vi "calcualte_scens.vi"(3 "Sort Scen":bool=TRUE, 5 "vy_in":T2(array[cluster])) -> (0 "boundaries":T1(array[cluster]), 2 "Scen out":T3(array[cluster]) {"xy_k_value" format="%#_3f"; "polygon" format="%#_3f"})   [LabVIEW 2011]
panel:
  out "scen_out":picture
  out "vy_in":picture
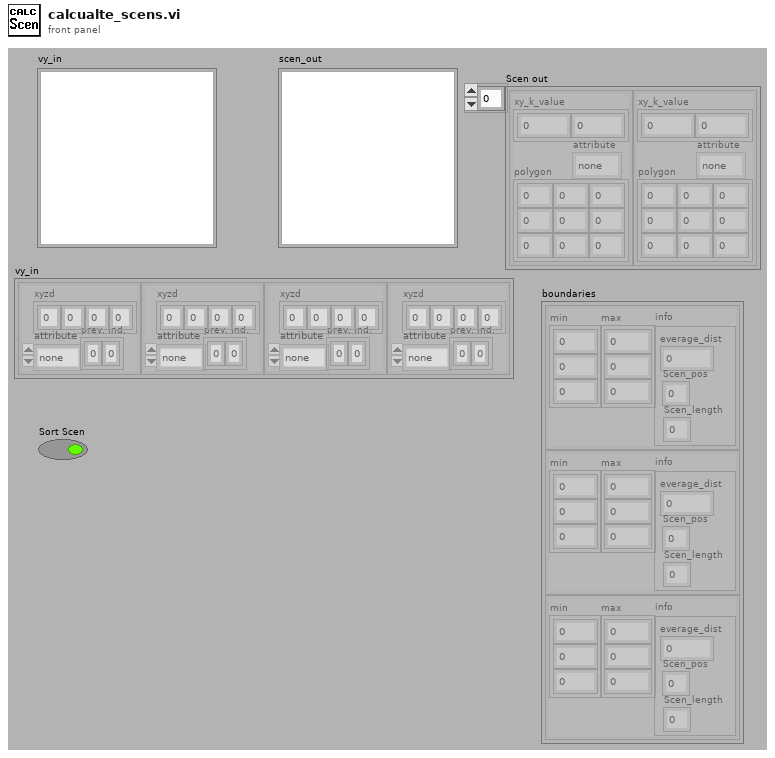
[diagram p1: front panel]
types:
  T1 = cluster{"min":dbl[], "max":dbl[], "info":cluster{"everage_dist":dbl, "Scen_pos":u16, "Scen_length":u16}}[]
  T2 = cluster{"xyzd":dbl[], "attribute":enum16{"none", "transparent", "reflective", "white", "black", "grey", "red", "yellow", "green", "blue", "pink"}, "prev. Ind.":i16[]}[]
  T3 = cluster{"xy_k_value":dbl[], "polygon":dbl[][], "attribute":enum16{"none", "transparent", "reflective", "white", "black", "grey", "red", "yellow", "green", "blue", "pink"}}[]
  T4 = cluster{"min":dbl[], "max":dbl[], "info":cluster{"everage_dist":dbl, "scen_pos":u16, "scen_length":u16}}
  T5 = cluster{"xy_k_value":dbl[], "polygon":dbl[][], "attribute":enum16{"none", "transparent", "reflective", "white", "black", "grey", "red", "yellow", "green", "blue", "pink"}}
  T6 = cluster{"min":dbl[], "max":dbl[], "info":cluster{"everage_dist":dbl, "scen_pos":u16, "scen_length":u16}}[]
  T7 = enum16{"none", "transparent", "reflective", "white", "black", "red", "yellow", "green", "blue", "pink"}
  T8 = enum16{"none", "transparent", "reflective", "white", "black", "grey", "red", "yellow", "green", "blue", "pink"}
  T9 = cluster{"xyzd":dbl[], "attribute":enum16{"none", "transparent", "reflective", "white", "black", "grey", "red", "yellow", "green", "blue", "pink"}, "prev. Ind.":i16[]}
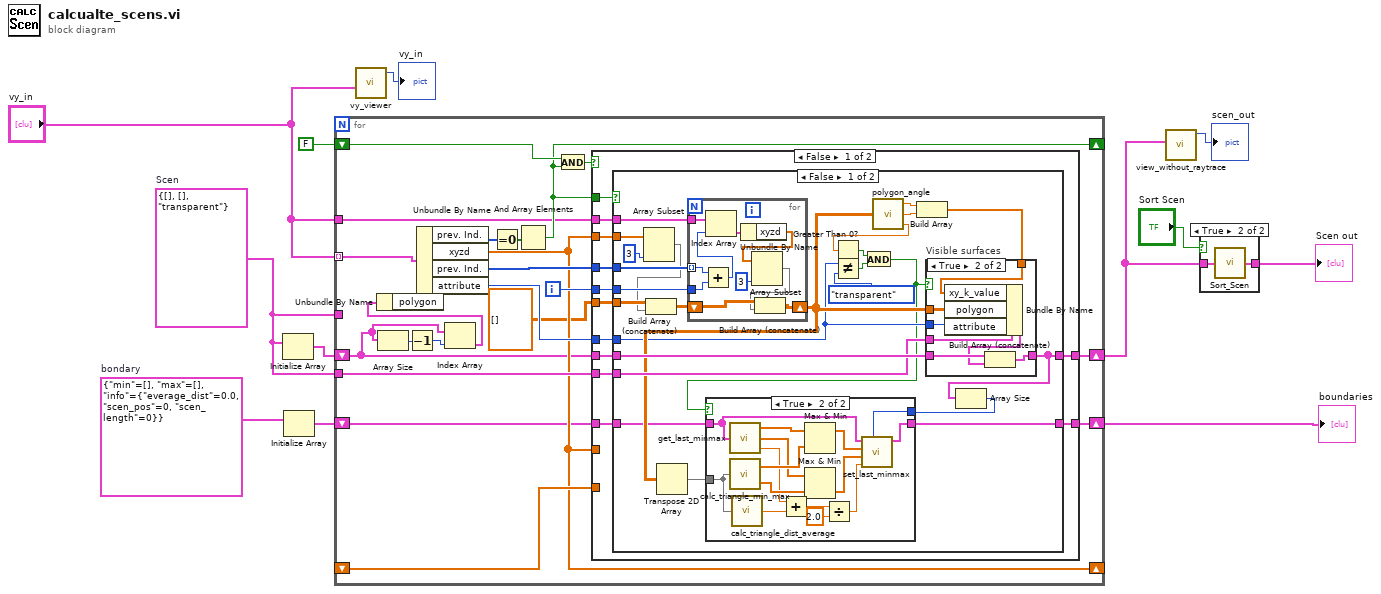
[diagram p0: block diagram]
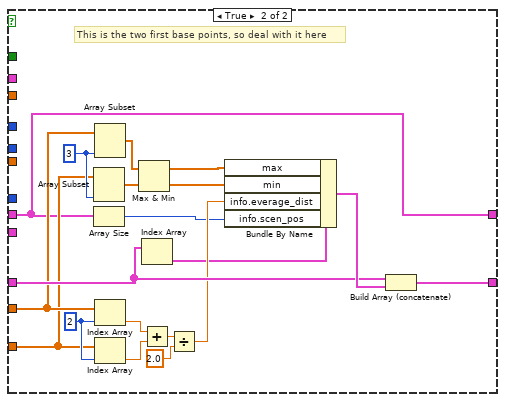
[diagram p6: hidden frame]
diagram:
  w6 = T4 {"min"=[], "max"=[], "info"={"everage_dist"=0.0, "scen_pos"=0, "scen_length"=0}}  # bondary
  w10 = T5 {"xy_k_value"=[], "polygon"=[], "attribute"=enum."transparent"}  # Scen
  n1 = Initialize Array(w10) -> (w9:T3)  [unwired: 1 in]
  n2 = Initialize Array(w6) -> (w7:T6)  [unwired: 1 in]
  n3 = for {
    tunnel: "vy_in" -> [w33] mode=indexing
    shift-right: [w13] -> w5
    shift-left: w7 -> [w14]
    shift-right: [w27] -> _
    shift-left: FALSE -> [w28]
    shift-right: [w18] -> _
    shift-left: _ -> [w29]
    shift-right: [w22] -> w2
    shift-left: w9 -> [w17]
    tunnel: "vy_in" -> [w24]
    tunnel: w10 -> [_]
    tunnel: w10 -> [w23]
    i -> [w25]
    n4 = Array Size(array=w17) -> (size(s)=w20:i32)
    n5 = Decrement(x=w20) -> (x-1=w19:i32)
    n6 = Unbundle By Name(w33) -> ("prev. Ind."=w32:i16[], "xyzd"=w18:dbl[], "prev. Ind."=w26:i16[], "attribute"=w21:T8)
    n7 = Index Array(array=w17, index=w19) -> (element=w16:T5)
    n8 = Unbundle By Name(w16) -> ()  [unwired: 1 out]
    n9 = Equal To 0?(x=w32) -> (x = 0?=w31:bool[])
    n10 = And Array Elements(Boolean array=w31) -> (logical AND=w27:bool)
    n11 = And(x=w28, y=w27) -> (x .and. y?=w30:bool)
    n12 = case shown="False" w30 {
      tunnel: w14 -> [w36 w114]
      tunnel: [w34 w109] -> w13
      tunnel: w18 -> [_ w113]
      tunnel: w29 -> [_ w111]
      tunnel: w27 -> [w45 _]
      tunnel: dbl[][] [] ("polygon") -> [w44 _]
      tunnel: w26 -> [w43 _]
      tunnel: w25 -> [w42 _]
      tunnel: w24 -> [w41 _]
      tunnel: w18 -> [w40 _]
      tunnel: w17 -> [w39 w108]
      tunnel: w23 -> [w38 _]
      tunnel: [w37 w108] -> w22
      tunnel: w21 -> [w35 _]
      frame False {
        n13 = case shown="False" w45 {
          tunnel: w44 -> [w60 _]
          tunnel: w43 -> [w70 _]
          tunnel: w42 -> [w69 _]
          tunnel: w41 -> [w68 _]
          tunnel: w40 -> [w61 _]
          tunnel: w39 -> [w66 w106]
          tunnel: w38 -> [w65 _]
          tunnel: [w55 w106] -> w37
          tunnel: w36 -> [w49 w105]
          tunnel: [w48 w105] -> w34
          tunnel: w35 -> [w51 _]
          frame False {
            n14 = Array Subset(array=w61, length=3) -> (w59:dbl[])  [unwired: 1 in]
            n15 = Build Array (concatenate)(w60, w59) -> (w58:dbl[][])
            n16 = for {
              tunnel: w70 -> [w104] mode=indexing
              tunnel: w69 -> [w103]
              tunnel: w68 -> [w102]
              shift-right: [w95] -> w57
              shift-left: w58 -> [w97]
              n17 = Add(x=w104, y=w103) -> (x+y=w100:i32)
              n18 = Index Array(array=w102, index=w100) -> (element=w101:T9)
              n19 = Unbundle By Name(w101) -> ("xyzd"=w98:dbl[])
              n20 = Array Subset(array=w98, length=3) -> (w96:dbl[])  [unwired: 1 in]
              n21 = Build Array (concatenate)(w97, w96) -> (w95:dbl[][])
            }
            n22 = Transpose 2D Array(2D array=w57) -> (transposed array=w56:dbl[][])
            n23 = Not Equal?(x=w51, y=T7."transparent") -> (x != y?=w52:bool)
            n24 = call "polygon_angle.vi"("polygon"=w57) -> ("kx"=w63:dbl, "ky"=w64:dbl, "z-angle"=w54:dbl)
            n25 = Greater Than 0?(x=w54) -> (x > 0?=w53:bool)
            n26 = And(x=w53, y=w52) -> (x .and. y?=w50:bool)
            n27 = Build Array(w63, w64) -> (w62:dbl[])
            n28 = case "Visible surfaces" shown="True" w50 {
              tunnel: w66 -> [w87 w94]
              tunnel: [w87 w93] -> w55
              tunnel: w65 -> [_ w92]
              tunnel: w57 -> [_ w90]
              tunnel: w62 -> [_ w89]
              tunnel: w51 -> [_ w88]
              frame False {
              }
              frame True {
                n29 = Bundle By Name(cluster=w92, "xy_k_value"=w89, "polygon"=w90, "attribute"=w88) -> (w91:T5)
                n30 = Build Array (concatenate)(w94, w91) -> (w93:T3)
              }
            }
            n31 = Array Size(array=w55) -> (size(s)=w47:i32)
            n32 = case shown="True" w50 {
              tunnel: w56 -> [_ w76]
              tunnel: w49 -> [w71 w75]
              tunnel: [w71 w74] -> w48
              tunnel: w47 -> [_ w73]
              frame False {
              }
              frame True {
                n33 = call "get_last_minmax.vi"("max_min_array"=w75) -> ("max_vector"=w86:dbl[], "min_vector"=w84:dbl[], "distance"=w79:dbl)
                n34 = call "calc_triangle_min_max.vi"("Array"=w76) -> ("Array 3"=w85:dbl[], "Array 2"=w83:dbl[])
                n35 = call "calc_triangle_dist_average.vi"("Array"=w76) -> ("Numeric"=w80:dbl)
                n36 = Add(x=w79, y=w80) -> (x+y=w78:dbl)
                n37 = Max & Min(x=w86, y=w85) -> (max(x,y)=w82:dbl[])  [unwired: 1 out]
                n38 = Max & Min(x=w84, y=w83) -> (min(x,y)=w81:dbl[])  [unwired: 1 out]
                n39 = Divide(x=w78, y=2.0) -> (x/y=w72:dbl)
                n40 = call "set_last_minmax.vi"("current_scen"=w73, "distance"=w72, "min_vector"=w81, "max_vector"=w82, "array_in"=w75) -> ("array_out"=w74:T6)  [unwired: 3 in]
              }
            }
          }
          frame True {
            # "This is the first base point, don't deal with it here"
          }
        }
      }
      frame True {
        w119 = 2 ("index")
        w121 = 3 ("length")
        # "This is the two first base points, so deal with it here"
        n41 = Array Subset(array=w111, length=w121) -> (w120:dbl[])  [unwired: 1 in]
        n42 = Array Size(array=w108) -> (size(s)=w107:i32)
        n43 = Array Subset(array=w113, length=w121) -> (w124:dbl[])  [unwired: 1 in]
        n44 = Index Array(array=w113, index=w119) -> (element=w122:dbl)
        n45 = Index Array(array=w111, index=w119) -> (element=w118:dbl)
        n46 = Max & Min(x=w124, y=w120) -> (max(x,y)=w123:dbl[], min(x,y)=w115:dbl[])
        n47 = Index Array(array=w114) -> (element=w110:T4)  [unwired: 1 in]
        n48 = Add(x=w122, y=w118) -> (x+y=w116:dbl)
        n49 = Divide(x=w116, y=2.0) -> (x/y=w112:dbl)
        n50 = Bundle By Name(cluster=w110, "max"=w123, "min"=w115, "info.everage_dist"=w112, "info.scen_pos"=w107) -> (w125:T4)
        n51 = Build Array (concatenate)(w114, w125) -> (w109:T6)
      }
    }
  }
  "boundaries" <- w5
  n52 = call "vy_viewer.vi"("vy_array"="vy_in") -> ("picture out"=→"vy_in":picture)  [unwired: 6 in]
  n53 = call "view_without_raytrace.vi"("Scens"=w2) -> ("new picture 2"=→"scen_out":picture)  [unwired: 8 in]
  n54 = case shown="True" "Sort Scen" {
    tunnel: [w126 w128] -> w12
    tunnel: w2 -> [w126 w127]
    frame False {
    }
    frame True {
      n55 = call "Sort_Scen.vi"("Scen in"=w127) -> ("Sorted Scen out"=w128:T3)
    }
  }
  "Scen out" <- w12
